vi "Read Abberation from Excel_SLM.vi"(6 "index":i32, 9 "Mode Matrices":path[](array[path])) -> (0 "Mode IDs":string[](array[string]), 3 "Mode":dbl[][](array[numeric]))   [LabVIEW 2018]
doc: "This example opens a worksheet in a specified Excel workbook and extracts data from the spreadsheet. The data can be interpreted either as numeric or string data, and the data can be in the form of a single cell of data or a 2D array.\n\nSelect an Excel workbook with the path control, specify a range of cells to read. Then go to\nthe block diagram and select the polymorphic instance corresponding to the type and range of data to read. You might have to recreate an indicator for the data if you change instances. Press run to extract the data from the Excel workbook."
panel:
  out "32bit integer":i32[](array[numeric])
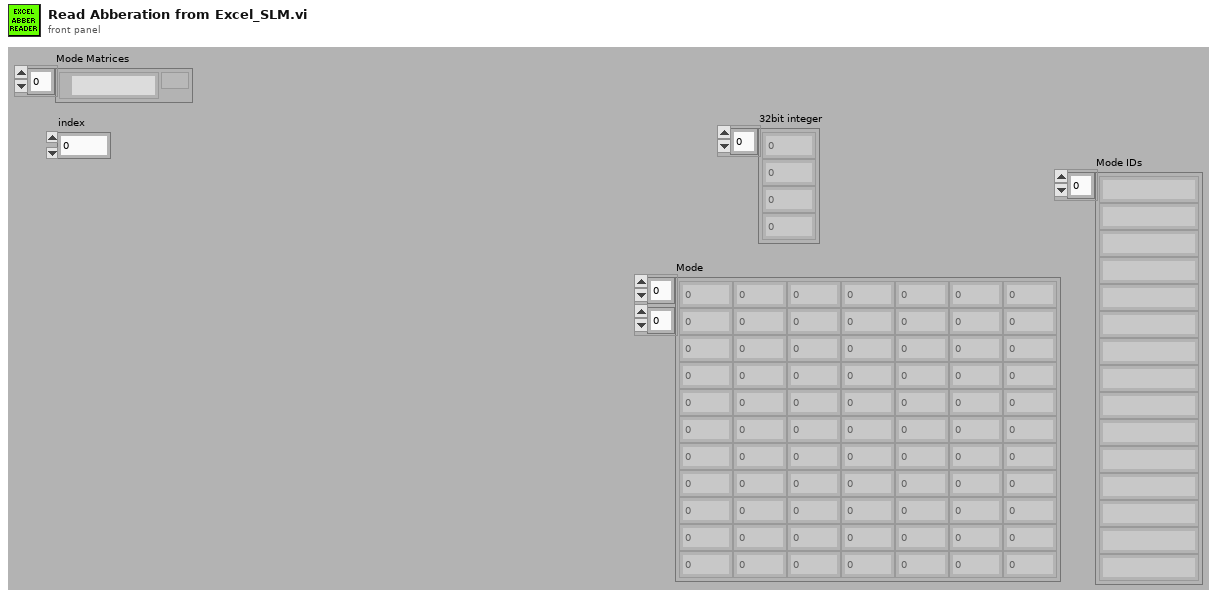
[diagram p1: front panel]
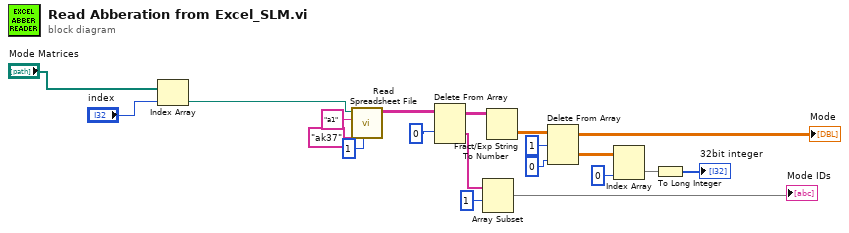
[diagram p0: block diagram]
diagram:
  n1 = Index Array(array="Mode Matrices", index="index") -> (element=w5:path)
  n2 = call "Read Spreadsheet File.vi"("Sheet No"=1, "End cell"="ak37", "Start Cell"="a1", "path"=w5) -> ("Array"=w2:string[][])  [unwired: 6 in, 1 out]
  n3 = Delete From Array(array=w2, index (row)=0 ("disabled index (col)")) -> (deleted portion=w18:string[], array with subset deleted=w20:string[][])  [unwired: 2 in]
  n4 = Array Subset(array=w18, index=1 ("length")) -> (→"Mode IDs":string[])  [unwired: 1 in]
  n5 = Fract/Exp String To Number(string=w20) -> (number=w16:dbl[][])  [unwired: 3 in, 1 out]
  n6 = Delete From Array(array=w16, length=1, index (col)=0 ("disabled index (col)")) -> (deleted portion=w13:dbl[][], array with subset deleted=→"Mode":dbl[][])  [unwired: 1 in]
  n7 = Index Array(array=w13, index (col)=0 ("disabled index (col)")) -> (element=w11:dbl[])  [unwired: 1 in]
  n8 = To Long Integer(number=w11) -> (32bit integer=→"32bit integer":i32[])
